vi "Organize Real Time Task Status.vi"(0 "Priority":i32, 1 "Processor":i32, 2 "Offset":i64, 3 "Iteration Duration":i64, 4 "Period":i64, 5 "Finished Late? [i-1]":bool, 8 "Task Name":string) -> (14 "Real Time Task Status":T1={"Task Name"="", "Priority"=100, "Processor"=-2, "Offset"=0, "Iteration Duration"=0, "Period"=0, "Finished Late"=FALSE})   [LabVIEW 2023]
uses:
  Type Definitions/Real Time Task Status.ctl
  Type Definitions/Enumerated Constants/Software Monitor.ctl
  Type Definitions/Payload Class.ctl
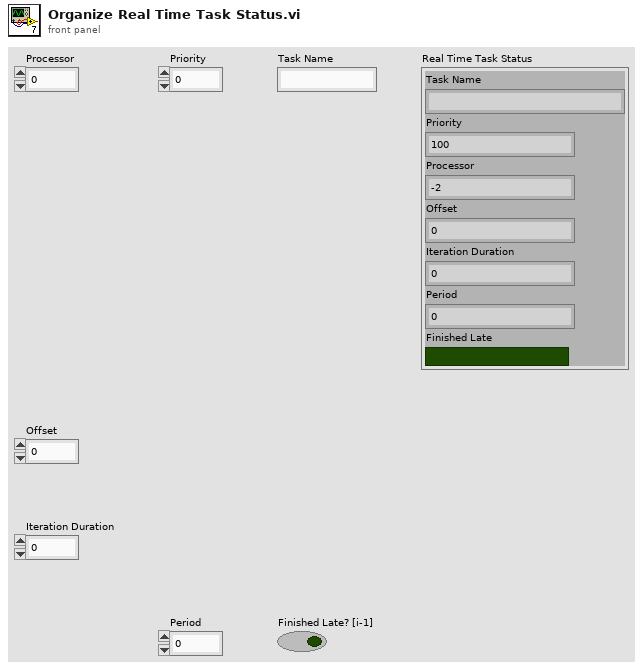
[diagram p1: front panel]
types:
  T1 = typedef "Real Time Task Status.ctl" = cluster{"Task Name":string, "Priority":i32, "Processor":i32, "Offset":i64, "Iteration Duration":i64, "Period":i64, "Finished Late":bool}
  T2 = typedef "Software Monitor.ctl" = enum16{"Internet Connection Monitor", "CPU Monitor", "Archive Monitor", "Memory Monitor", "Queue Monitor", "RTOS Update", "RTOS Monitor"}
  T3 = typedef "Payload Class.ctl" = enum16{"System State", "Parameters", "Metadata", "Software Monitor", "Data", "Commands"}
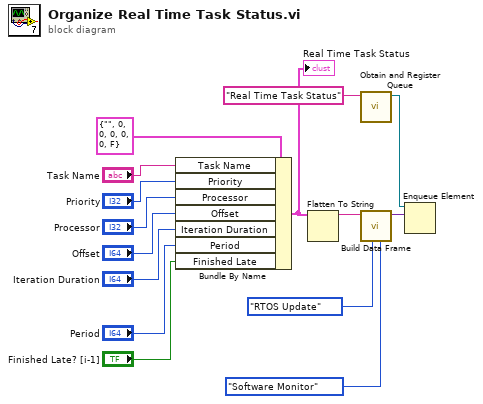
[diagram p0: block diagram]
diagram:
  n1 = Bundle By Name(cluster=T1 {"Task Name"="", "Priority"=0, "Processor"=0, "Offset"=0, "Iteration Duration"=0, "Period"=0, "Finished Late"=FALSE} ("Cluster"), "Task Name"="Task Name", "Priority"="Priority", "Processor"="Processor", "Offset"="Offset", "Iteration Duration"="Iteration Duration", "Period"="Period", "Finished Late"="Finished Late? [i-1]") -> (w7:T1)
  "Real Time Task Status" <- w7
  n2 = Flatten To String(anything=w7) -> (data string=w5:string)  [unwired: 3 in, 2 out]
  n3 = call "Obtain and Register Queue.vi"("Queue Name (unnamed)"="Real Time Task Status" ("name (unnamed)")) -> ("Queue Reference"=w8:refnum<queue>)  [unwired: 9 in, 1 out]
  n4 = call "Build Data Frame.vi"("Payload Class (Data)"=Payload_Class."Software Monitor", "Payload ID (0)"=Software_Monitor."RTOS Update", "Payload (Empty String)"=w5) -> ("Frame"=w6:variant)  [unwired: 7 in, 1 out]
  n5 = Enqueue Element(queue=w8, element=w6) -> ()  [unwired: 2 in, 3 out]
